vi "_Yt03_ELSE IF.vi"(11 "YTESTER测试数据":T1) -> (3 "YTESTER结论":T2)   [LabVIEW 2017]
doc: "VIClassID=YT_SSTEPFLAG_ELSEIF\nVIDescription=否则如果"
uses:
  YtCommon.lvlibp/yt`Step StepBaseInput.ctl
  Step`s VIs/YYLLIdea/yylltestresult/yylltestresult basis.ctl
  YtCommon.lvlibp/yt`Step StepResult.ctl
  YtCommon.lvlibp/yt`Step TestData.ctl
  YtCommon.lvlibp/yt`Step System Queue.ctl
  YtCommon.lvlibp
panel:
  in  "YTESTER开放参数":T5={"YTESTER_BaseInput"={"isTest"=FALSE, "isSkip"=FALSE, "StepName"="Else If", "OnPass"=enum."Next", "OnFail"=enum."Next", "ReTestNumber"=0.0}, "Smart预处理"=[], "数据源什么类型？"=enum."String类型", "String数据源"="", "NUM数据源"=0.0, "Bool数据源"=FALSE, "合格依据"=enum."强制合格", "StringLimit-A"="", "UpperLimit-B"=0.0, "LowLimit-C"=0.0, "unit"=""}
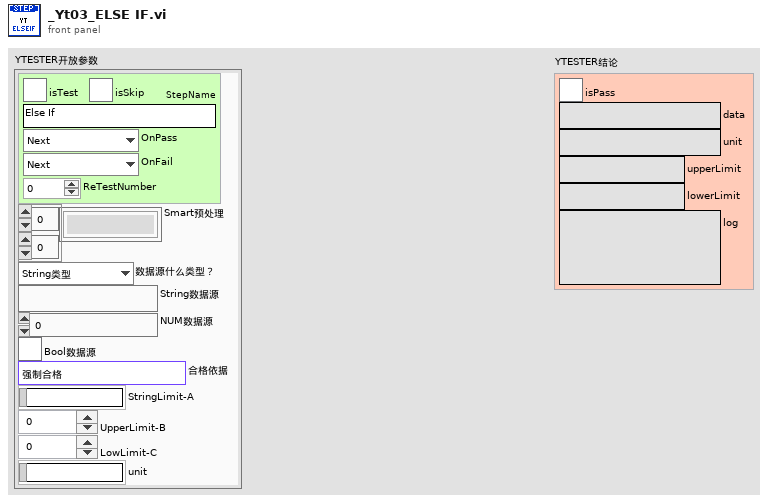
[diagram p1: front panel]
types:
  T1 = typedef "YtCommon.lvlibp/yt`Step TestData.ctl" = cluster{"Socket(From1)":i32, "SN":refnum<notifier>, "StopFlagRef":refnum<notifier>, "YT System Queue":refnum<queue>}
  T2 = typedef "YtCommon.lvlibp/yt`Step StepResult.ctl" = cluster{"isPass":bool, "data":string, "unit":string, "upperLimit":string, "lowerLimit":string, "log":string}
  T3 = typedef "YtCommon.lvlibp/yt`Step StepBaseInput.ctl" = cluster{"isTest":bool, "isSkip":bool, "StepName":string, "OnPass":enum16{"Next", "ToOVER", "Terminate"}, "OnFail":enum16{"Next", "ToOVER", "Terminate"}, "ReTestNumber":dbl}
  T4 = typedef "yylltestresult basis.ctl" = enum16{"强制合格", "强制不合格", "随机合格", "X=A", "X=\"真\"", "X=\"假\"", "X≠A", "X包含A", "X不包含A", "A包含X", "A包含非空X", "A不包含X", "X等于A正则匹配内容", "X包含A正则匹配内容", "X不包含A正则匹配内容", "X=B", "X≠B", "X＞B", "X≥B", "X＜B", "X≤B", "B≥X≥C", "B≥X＞C", "B＞X≥C", "B＞X＞C", "X≥B | C≥X", "X＞B | C≥X", "X≥B | C＞X", "X＞B | C＞X"}
  T5 = cluster{"YTESTER_BaseInput":T3, "Smart预处理":string[][], "数据源什么类型？":enum16{"String类型", "NUM类型", "Bool类型"}, "String数据源":string, "NUM数据源":dbl, "Bool数据源":bool, "合格依据":T4, "StringLimit-A":string, "UpperLimit-B":dbl, "LowLimit-C":dbl, "unit":string}
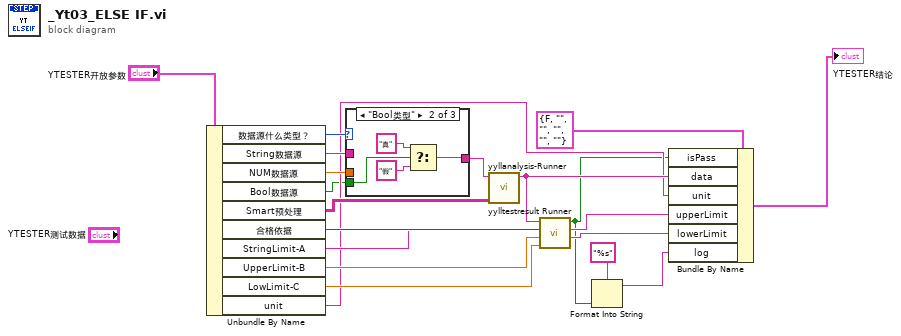
[diagram p0: block diagram]
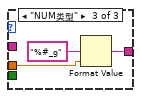
[diagram p3: hidden frame]
diagram:
  n1 = Unbundle By Name("YTESTER开放参数") -> ("数据源什么类型？"=w19:enum16{"String类型", "NUM类型", "Bool类型"}, "String数据源"=w18:string, "NUM数据源"=w17:dbl, "Bool数据源"=w1:bool, "Smart预处理"=w15:string[][], "合格依据"=w14:T4, "StringLimit-A"=w13:string, "UpperLimit-B"=w12:dbl, "LowLimit-C"=w11:dbl, "unit"=w9:string)
  n2 = case shown="\"Bool类型\"" w19 {
    tunnel: w18 -> [w21 _ _]
    tunnel: [w21 w22 w27] -> w16
    tunnel: w17 -> [_ _ w28]
    tunnel: w1 -> [_ w23 _]
    frame "String类型" {
    }
    frame "Bool类型" {
      n3 = Select(t="真", s=w23, f="假") -> (s? t:f=w22:string)
    }
    frame "NUM类型" {
      n4 = Format Value(format string="%#_g", value (0)=w28) -> (output string=w27:string)  [unwired: 1 in]
    }
  }
  n5 = call "yyllanalysis-Runner.vi"("inputs"=w15, "String in"=w16) -> ("String out"=w10:string)  [unwired: 8 in, 1 out]
  n6 = call "yylltestresult Runner.vi"("合格依据"=w14, "LowLimit-C"=w11, "UpperLimit-B"=w12, "StringLimit-A"=w13, "DataIn-X"=w10) -> ("lowerLimit"=w7:string, "upperLimit"=w8:string, "isPass"=w6:bool)  [unwired: 4 in]
  n7 = Format Into String(format string="%s", w6) -> (resulting string=w4:string)  [unwired: 2 in, 1 out]
  n8 = Bundle By Name(cluster=T2 {"isPass"=FALSE, "data"="", "unit"="", "upperLimit"="", "lowerLimit"="", "log"=""} ("Result"), "isPass"=w6, "data"=w10, "unit"=w9, "upperLimit"=w8, "lowerLimit"=w7, "log"=w4) -> (→"YTESTER结论":T2)
